vi "DataLog Read Log Index Range.vi"(0 "tag log directory":path, 7 "log index":dbl, 9 "number of points":i32, 11 "error in (no error)":errorcluster) -> (4 "dup tag log directory":path, 8 "range of points":T1[](array[typedef]) {"value" format="%.3e"; "time" format="%<%H:%M:%S%2u\n%Y/%m/%d>T"}, 15 "error out":errorcluster)   [LabVIEW 2012]
doc: "Read the range of points starting at the specified index from a tag's log."
uses:
  typedefs/clusters/t_DataLog Point.ctl
  private/glb_DataLog Runtime Parameterisation.vi
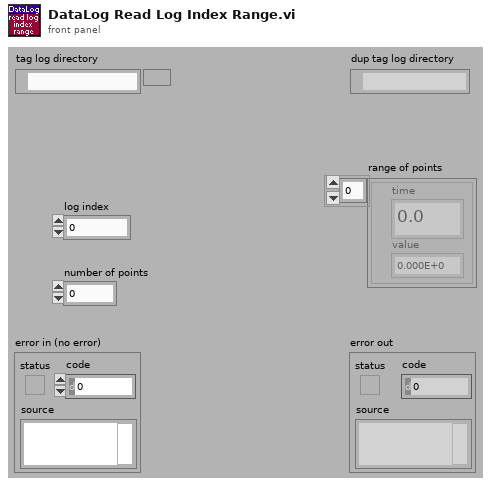
[diagram p1: front panel]
types:
  T1 = typedef "t_DataLog Point.ctl" = cluster{"time":dbl, "value":dbl}
  T2 = enum16{"read/write", "read-only", "write-only", "write-only (truncate)"}
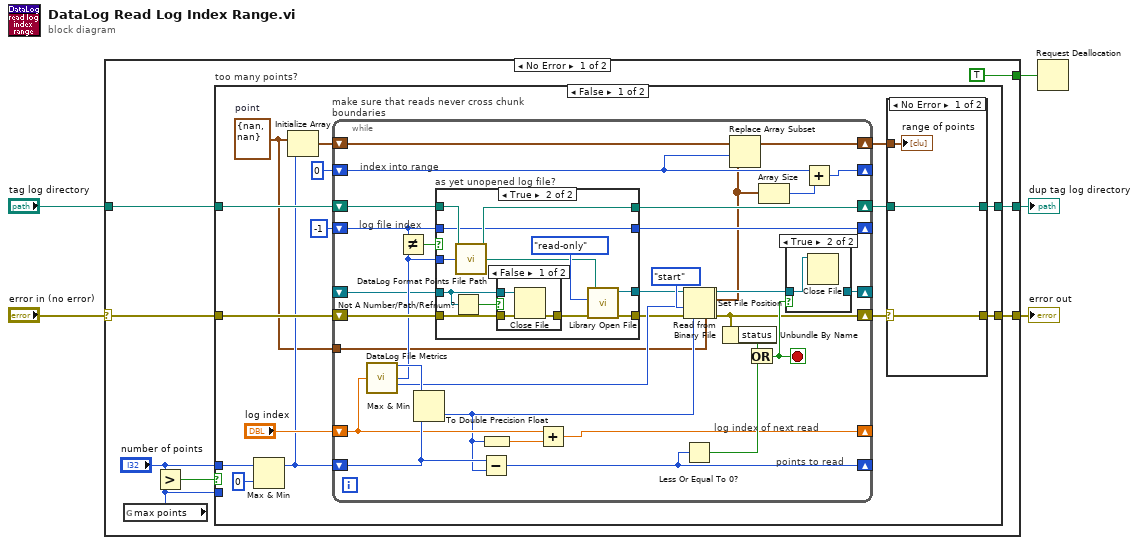
[diagram p0: block diagram]
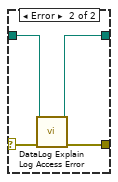
[diagram p2: hidden frame]
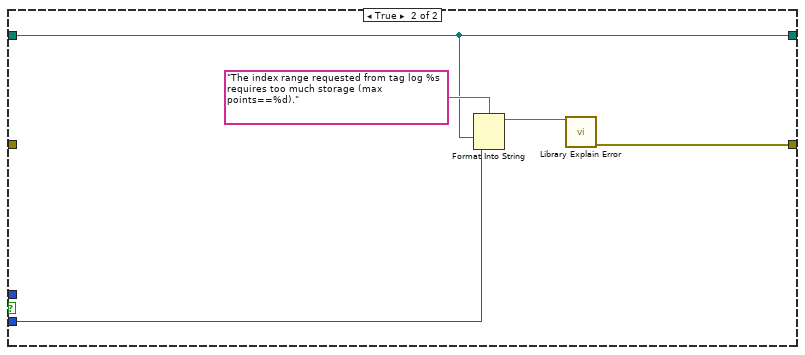
[diagram p6: hidden frame]
diagram:
  n1 = case shown="No Error" "error in (no error)" {
    selector: "error in (no error)" -> [w10 w97]
    tunnel: [w13 w97] -> w5
    tunnel: "tag log directory" -> [w11 w96]
    tunnel: [w12 w96] -> w2
    tunnel: [TRUE _] -> w1
    frame No Error {
      n2 = global read "glb_DataLog Runtime Parameterisation.vi" "max points"() -> (w7:i32)
      n3 = Greater?(x="number of points", y=w7) -> (0:w8:bool)
      n4 = case "too many points?" shown="False" w8 {
        tunnel: [w28 w91] -> w13
        tunnel: [w27 w92] -> w12
        tunnel: w11 -> [w26 w92]
        tunnel: w10 -> [w24 _]
        tunnel: "number of points" -> [w14 _]
        tunnel: w7 -> [_ w93]
        frame False {
          w15 = T1 {"time"=nan, "value"=nan}  # point
          n5 = Max & Min(x=w14, y=0) -> (max(x,y)=w19:i32)  [unwired: 1 out]
          n6 = Initialize Array(w15, w19) -> (w16:T1[])
          n7 = while "make sure that reads never cross chunk boundaries" {
            shift-right: [w57] -> w25
            shift-left: w26 -> [w68]
            shift-right: [w45] -> w22
            shift-left: w24 -> [w63]
            shift-right: [w65] -> _
            shift-left: w19 -> [w66]
            shift-right: [w59] -> _
            shift-left: "log index" -> [w61]
            shift-right: [w52] -> _
            shift-left: -1 ("log file index") -> [w53]
            shift-right: [w55] -> _
            shift-left: _ -> [w51]
            shift-right: [w43] -> w17
            shift-left: w16 -> [w44]
            shift-right: [w41] -> _
            shift-left: 0 ("log file index") -> [w42]
            tunnel: w15 -> [w38]
            stop <- w56 stop-if-true
            # "log file index"
            # "points to read"
            # "log index of next read"
            # "index into range"
            n8 = call "DataLog File Metrics.vi"("point index"=w61) -> ("points left in chunk"=w67:i32, "log file index"=w58:i32, "log file offset"=w47:i32)  [unwired: 9 in, 3 out]
            n9 = Not Equal?(x=w53, y=w58) -> (x != y?=w54:bool)
            n10 = Max & Min(x=w67, y=w66) -> (min(x,y)=w46:i32)  [unwired: 1 out]
            n11 = case "as yet unopened log file?" shown="True" w54 {
              tunnel: w68 -> [w71 w84]
              tunnel: w63 -> [w69 w76]
              tunnel: [w69 w82] -> w45
              tunnel: w58 -> [_ w81]
              tunnel: [w71 w80] -> w57
              tunnel: [w70 w78] -> w49
              tunnel: w53 -> [w72 w77]
              tunnel: [w72 w77] -> w52
              tunnel: w51 -> [w70 w75]
              frame False {
              }
              frame True {
                n12 = Not A Number/Path/Refnum?(number/path/refnum=w75) -> (NaN/Path/Refnum?=w74:bool)
                n13 = call "DataLog Format Points File Path.vi"("tag log directory"=w84, "log file index"=w81) -> ("dup tag log directory"=w80:path, "log file path"=w79:path)  [unwired: 12 in]
                n14 = case shown="False" w74 {
                  tunnel: w76 -> [w87 w88]
                  tunnel: w75 -> [w86 _]
                  tunnel: [w85 w88] -> w73
                  frame False {
                    n15 = Close File(refnum=w86, error in=w87) -> (error out=w85:errorcluster)  [unwired: 1 out]
                  }
                  frame True {
                  }
                }
                n16 = call "Library Open File.vi"("error in (no error)"=w73, "open mode (read/write)"=T2."read-only" ("open mode (0)"), "file path"=w79) -> ("error out"=w82:errorcluster, "refnum"=w78:refnum<file>)  [unwired: 3 in]
              }
            }
            n17 = Subtract(x=w66, y=w46) -> (x-y=w65:i32)
            n18 = To Double Precision Float(number=w46) -> (double precision float=w60:dbl)
            n19 = Add(x=w61, y=w60) -> (x+y=w59:dbl)
            n20 = Set File Position(offset (in bytes) (0)=w47, refnum=w49, from (0:start)=enum16{"start", "end", "current"}."start" ("pos mode (0:2)")) -> (refnum out=w37:refnum<file>, error out=w36:errorcluster)  [unwired: 1 in]
            n21 = Less Or Equal To 0?(x=w65) -> (x <= 0?=w64:bool)
            n22 = Read from Binary File(5:w38, 8:w36, 10:w46, 11:w37) -> (2:w39:T1[], 3:w48:refnum<file>)  [unwired: 2 in, 2 out]
            n23 = Unbundle By Name(w45) -> ("status"=w62:bool)
            n24 = Replace Array Subset(array=w44, new element=w39, index=w42) -> (w43:T1[])
            n25 = Or(x=w62, y=w64) -> (x .or. y?=w56:bool)
            n26 = Array Size(array=w39) -> (size(s)=w40:i32)
            n27 = case shown="True" w56 {
              tunnel: w48 -> [w89 w90]
              tunnel: [w89 _] -> w55
              frame False {
              }
              frame True {
                n28 = Close File(refnum=w90) -> ()  [unwired: 1 in, 2 out]
              }
            }
            n29 = Add(x=w42, y=w40) -> (x+y=w41:i32)
          }
          n30 = case shown="No Error" w22 {
            selector: w22 -> [w30 w34]
            tunnel: [w30 w35] -> w28
            tunnel: w25 -> [w31 w33]
            tunnel: [w31 w32] -> w27
            tunnel: w17 -> [w29 _]
            frame No Error {
              "range of points" <- w29
            }
            frame Error {
              n31 = call "DataLog Explain Log Access Error.vi"("tag log directory"=w33, "error in"=w34) -> ("dup tag log directory"=w32:path, "error out"=w35:errorcluster)  [unwired: 12 in]
            }
          }
        }
        frame True {
          n32 = Format Into String(format string="The index range requested from tag log %s requires too much storage (max points==%d).", w92, w93) -> (resulting string=w95:string)  [unwired: 2 in, 1 out]
          n33 = call "Library Explain Error.vi"("explanation prefix (none)"=w95) -> ("explained error"=w91:errorcluster)  [unwired: 14 in]
        }
      }
    }
    frame Error {
    }
  }
  "error out" <- w5
  "dup tag log directory" <- w2
  n34 = Request Deallocation(w1) -> ()
